vi "Test Thermal Chamber Simulator AE.vi"() -> ()   [LabVIEW 2015, in "Thermal Chamber Response Simulator.lvlib"]
doc: "Tester VI for the thermal chamber simulator Action Engine (AE).\n____\nDelacor QMH Thermal Chamber Examples 4.0.0.21\nCopyright (c) 2018, Delacor"
uses:
  Thermal Chamber Response Simulator.lvlib
  Action--enum.ctl
panel:
  in  "Ramp Rate (deg C / second)":dbl=1.0
  in  "Temperature Set Point (deg C)":dbl
  in  "Furnace Function":T1
  out "Furnace Temperature Chart":dbl(graph)
  out "Shut Down Furnace?":bool
  out "Required Temperature deg C":dbl
  out "Ramp Rate deg C/second":dbl
  out "Furnace Temperature":dbl
  in  "stop":bool
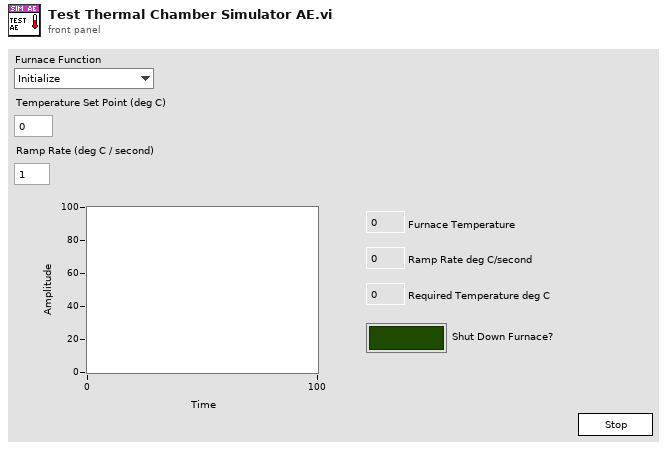
[diagram p1: front panel]
types:
  T1 = typedef "Thermal Chamber Response Simulator.lvlib/Action--enum.ctl" = enum16{"Initialize", "Set Temperature Required", "Set Ramp Rate", "Get Status", "Disable Heater", "Enable Heater", "Exit Application"}
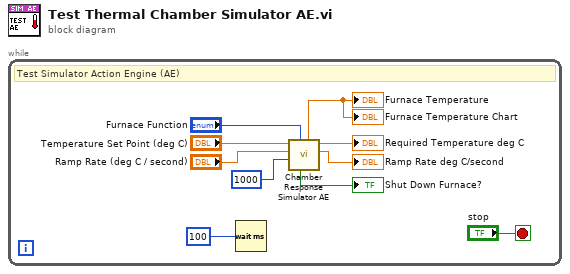
[diagram p0: block diagram]
diagram:
  n1 = while {
    stop <- "stop" stop-if-true
    # "Test Simulator Action Engine (AE)"
    n2 = Wait (ms)(milliseconds to wait=u32 100 ("millisecond multiple")) -> ()  [unwired: 1 out]
    n3 = call "Chamber Response Simulator AE.vi"("Thermal Chamber Function"="Furnace Function", "Time Interval (ms)"=u32 1000, "Ramp Rate in"="Ramp Rate (deg C / second)", "Temperature Set Point in"="Temperature Set Point (deg C)") -> ("Ramp Rate out"=→"Ramp Rate deg C/second":dbl, "Temperature Set Point out"=→"Required Temperature deg C":dbl, "Actual Temperature"=→"Furnace Temperature" →"Furnace Temperature Chart":dbl, "Shutdown Furnace?"=→"Shut Down Furnace?":bool)  [unwired: 2 in, 2 out]
  }
